vi "Delete Item.vi"(0 "Data In in":T1 caption="Data In", 2 "LstBox Refnum":refnum<vi>, 7 "Display State In":T2) -> (4 "Data In out":T1 caption="Data In")   [LabVIEW 2020, in "KListbox.xctl"]
uses:
  KListbox.xctl
  State.ctl
  Events.ctl
  Event Action.ctl
  Data.ctl
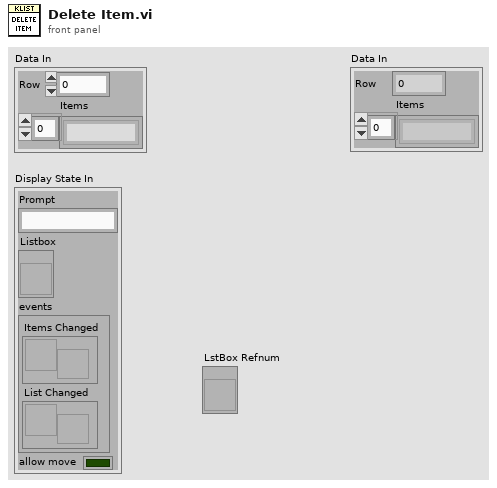
[diagram p1: front panel]
types:
  T1 = typedef "KListbox.xctl/Data.ctl" = cluster{"Row":i32, "Items":string[]}
  T2 = typedef "KListbox.xctl/State.ctl" = cluster{"Prompt":string, "Listbox":refnum<vi>, "events":T3, "allow move":bool}
  T3 = typedef "KListbox.xctl/Events.ctl" = cluster{"Items Changed":refnum<user-event>, "List Changed":refnum<user-event>}
  T4 = typedef "KListbox.xctl/Event Action.ctl" = enum16{"Select", "Add", "Delete", "Edit"}
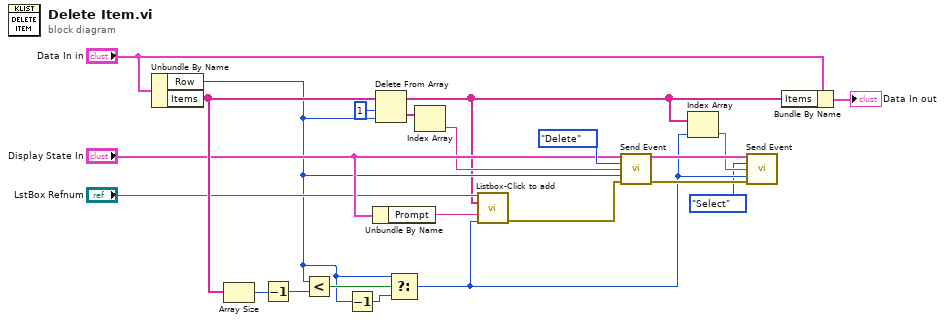
[diagram p0: block diagram]
diagram:
  n1 = Unbundle By Name("Data In in") -> ("Row"=w5:i32, "Items"=w19:string[])
  n2 = Array Size(array=w19) -> (size(s)=w22:i32)
  n3 = Decrement(x=w22) -> (x-1=w13:i32)
  n4 = Less?(x=w5, y=w13) -> (x < y?=w15:bool)
  n5 = Decrement(x=w5) -> (x-1=w14:i32)
  n6 = Unbundle By Name("Display State In") -> ("Prompt"=w12:string)
  n7 = Delete From Array(array=w19, length=1, index=w5) -> (deleted portion=w16:string[], array with subset deleted=w4:string[])
  n8 = Select(t=w5, s=w15, f=w14) -> (s? t:f=w3:i32)
  n9 = Index Array(array=w16) -> (element=w6:string)  [unwired: 1 in]
  n10 = call "Listbox-Click to add.vi"("ListBox"="LstBox Refnum", "Strings"=w4, "Prompt"=w12, "Row"=w3) -> ("error out"=w9:errorcluster)  [unwired: 10 in, 1 out]
  n11 = call "Send Event.vi"("State"="Display State In", "action"=Event_Action."Delete", "Name"=w6, "Row"=w5, "error in (no error)"=w9) -> ("State thru"=w7:T2, "error out"=w8:errorcluster)  [unwired: 9 in]
  n12 = Index Array(array=w4, index=w3) -> (element=w2:string)
  n13 = call "Send Event.vi"("State"=w7, "action"=Event_Action."Select", "Name"=w2, "Row"=w3, "error in (no error)"=w8) -> ()  [unwired: 9 in, 2 out]
  n14 = Bundle By Name(cluster="Data In in", "Items"=w4) -> (→"Data In out":T1)
